vi "Main Page.vi"(8 "error in (no error)":errorcluster, 11 "Node Ptr":T1 format="%.0x") -> (0 "error out":errorcluster)   [LabVIEW 2019, in "FPGA Addon System Explorer.lvlib"]
uses:
  FPGA Addon System Explorer.lvlib
  <vilib>/NI VeriStand/Custom Device API/Custom Device API.lvlib
  Addon Shared/FPGA Addon Shared.lvlib
  Addon Shared/Types/FG Action.ctl
  <vilib>/NI/NI VeriStand Hardware Resource Discovery/NIVS Hardware Discovery.lvlib
  <vilib>/NI/NI VeriStand Hardware Resource Discovery/_Types/Filter Type.ctl
  <vilib>/NI VeriStand/Custom Device API/Custom Device Item Ref.ctl
panel:
  in  "RIO Browse":bool
  out "Version":string
  in  "SHDocVw.IWebBrowser":refnum<k7>(container)
  in  "RIO Device":string
  in  "Bitfile path":path
  in  "Header 2":cluster{"Section Name":string}={"Section Name"="Custom Device Item Settings"}
  in  "Header":cluster{"Section Name":string}={"Section Name"="Custom Device Item Settings"}
  in  "Description":string
  in  "Name":string
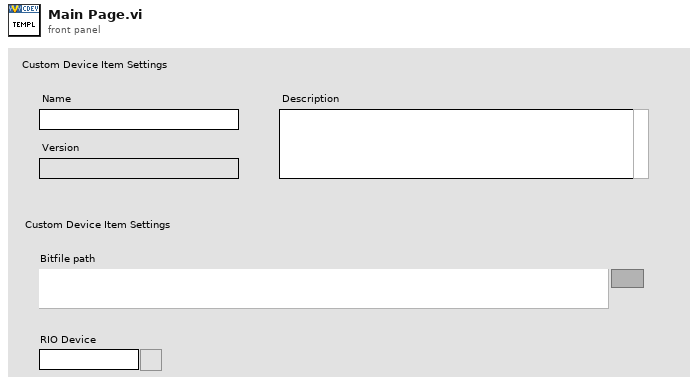
[diagram p1: front panel]
types:
  T1 = typedef "Custom Device API.lvlib/Custom Device Item Ref.ctl" = u64
  T2 = typedef "FPGA Addon Shared.lvlib/FG Action.ctl" = enum8{"GET", "SET"}
  T3 = typedef "FPGA Addon Shared.lvlib/FPGA Settings.ctl" = cluster{"Bitfile path":path, "RIO Device Address":string}
  T4 = typedef "Custom Device API.lvlib/Custom Device Item Info.ctl" = cluster{"Name":string, "Is Channel":bool, "GUID":string, "Is Waveform":bool}
  T5 = typedef "NIVS Hardware Discovery.lvlib/Filter Type.ctl" = enum16{"Device Category", "Product Name", "Ethernet", "XNET", "VISA", "FPGA", "EtherCAT Master", "DAQmx", "GPIB", "Serial"}
  T6 = typedef "Custom Device API.lvlib/Custom Device Commands.ctl" = enum16{"Default", "Item renamed", "Shutdown", "Dynamic button pressed"}
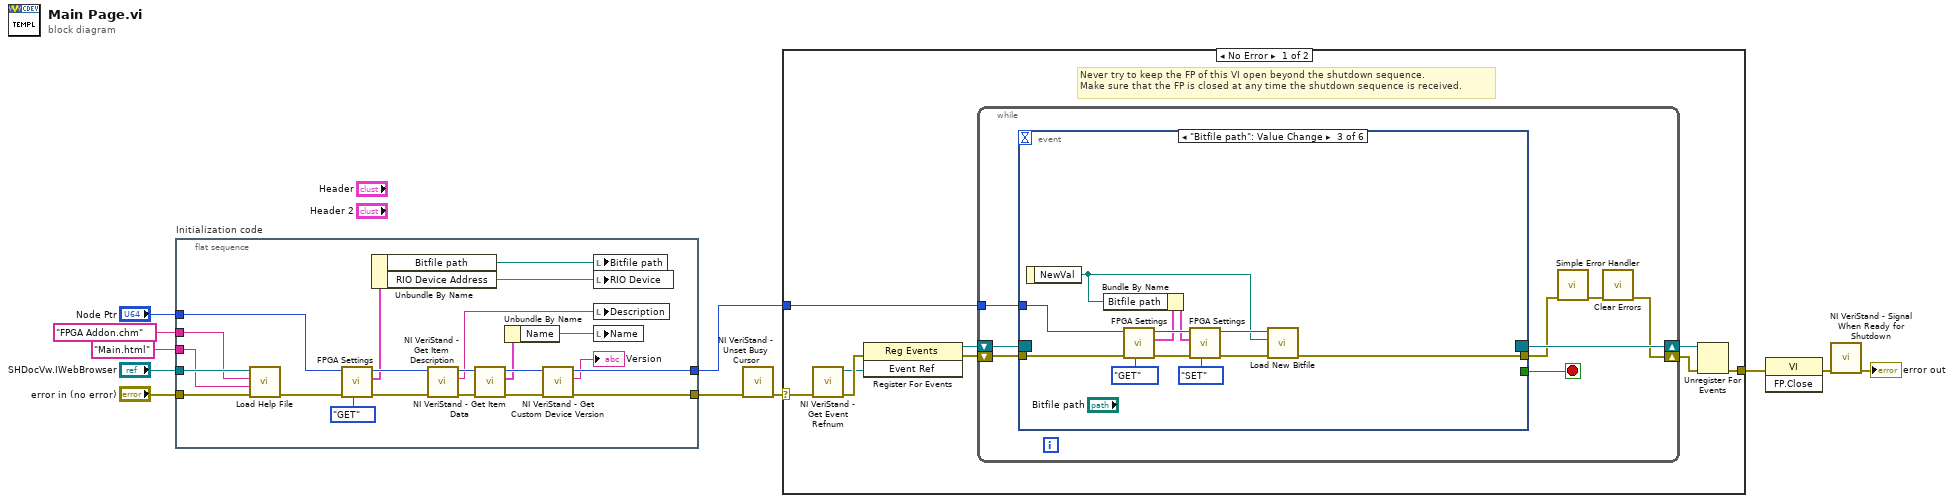
[diagram p0: block diagram]
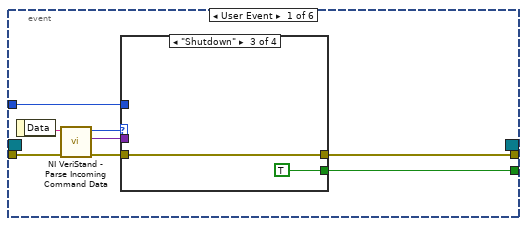
[diagram p2: hidden frame]
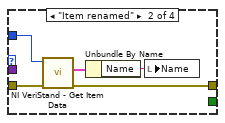
[diagram p4: hidden frame]
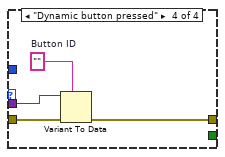
[diagram p5: hidden frame]
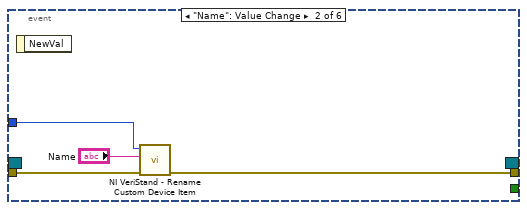
[diagram p6: hidden frame]
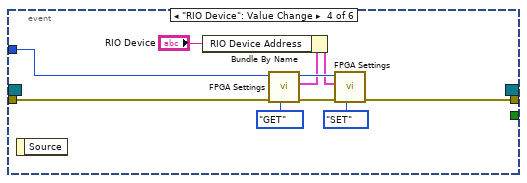
[diagram p7: hidden frame]
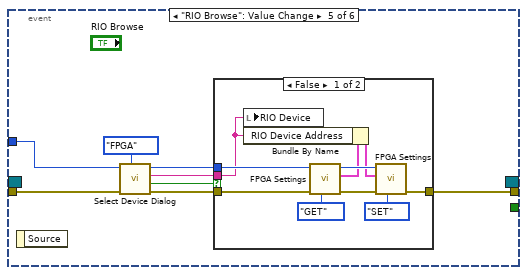
[diagram p8: hidden frame]
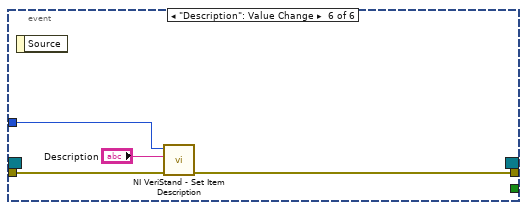
[diagram p10: hidden frame]
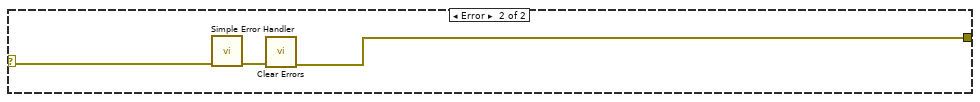
[diagram p11: hidden frame]
diagram:
  n1 = flat-sequence "Initialization code" {
    tunnel: "error in (no error)" -> [w27]
    tunnel: "Node Ptr" -> [w23]
    tunnel: [w14] -> w7
    tunnel: [w15] -> w4
    tunnel: "SHDocVw.IWebBrowser" -> [w26]
    tunnel: "Main.html" ("HTML File") -> [w25]
    tunnel: "FPGA Addon.chm" ("Main CHM File") -> [w24]
    frame #0 {
      n2 = call "Load Help File.vi"("error in (no error)"=w27, "HTML File"=w25, "Main CHM File"=w24, "SHDocVw.IWebBrowser2"=w26) -> ("error out"=w22:errorcluster)  [unwired: 7 in]
      n3 = call "FPGA Settings.vi"("Action"=FG_Action."GET", "error in (no error)"=w22, "Item Ref"=w23) -> ("error out"=w20:errorcluster, "FPGA Settings"=w18:T3, "Item Ref out"=w21:T1)  [unwired: 6 in]
      n4 = Unbundle By Name(w18) -> ("Bitfile path"=w16:path, "RIO Device Address"=w17:string)
      n5 = call <vilib>:"NI VeriStand - Get Item Description.vi"("error in (no error)"=w20, "Item Ref in"=w21) -> ("error out"=w30:errorcluster, "Description"=w31:string, "Item Ref out"=w32:T1)  [unwired: 7 out]
      n6 = call <vilib>:"NI VeriStand - Get Item Data.vi"("error in (no error)"=w30, "Item Ref in"=w32) -> ("error out"=w13:errorcluster, "Item Info"=w29:T4, "Item Ref out"=w33:T1)  [unwired: 7 out]
      n7 = Unbundle By Name(w29) -> ("Name"=w28:string)
      n8 = call <vilib>:"NI VeriStand - Get Custom Device Version.vi"("error in (no error)"=w13, "Device Ref in"=w33) -> ("error out"=w14:errorcluster, "Value"=→"Version":string, "Device Ref out"=w15:T1)  [unwired: 7 in]
      n9 = local write "Bitfile path"(w16) -> ()
      n10 = local write "RIO Device"(w17) -> ()
      n11 = local write "Description"(w31) -> ()
      n12 = local write "Name"(w28) -> ()
    }
  }
  n13 = call <vilib>:"NI VeriStand - Unset Busy Cursor.vi"("error in (no error)"=w7) -> ("error out"=w6:errorcluster)  [unwired: 10 out]
  n14 = case shown="No Error" w6 {
    selector: w6 -> [w34 w122]
    tunnel: [w39 w120] -> w11
    tunnel: w4 -> [w35 _]
    frame No Error {
      # "Never try to keep the FP of this VI open beyond the shutdown sequence.\nMake sure that the FP is closed at any time the shutdown sequence is received."
      n15 = call <vilib>:"NI VeriStand - Get Event Refnum.vi"("error in (no error)"=w34) -> ("error out"=w42:errorcluster, "Event Ref"=w38:refnum<user-event>)  [unwired: 9 out]
      n16 = register-events(error in=w42, w38) -> (reference out=w36:refnum<event-registration>, error out=w37:errorcluster)  [unwired: 1 in]
      n17 = while {
        tunnel: w35 -> [w46]
        shift-right: [w43] -> w40
        shift-left: w37 -> [w49]
        shift-right: [w50] -> w41
        shift-left: w36 -> [w48]
        stop <- w47 stop-if-true
        n18 = event shown="[2] \"Bitfile path\": Value Change" {
          selector: w48 -> [_ _ _ _ _ _]
          dyn-events: [_ _ _ _ _ _] -> w50
          timeout: _ -> [_ _ _ _ _ _]
          tunnel: w49 -> [w58 w74 w81 w90 w102 w118]
          tunnel: [w54 _ _ _ _ _] -> w47
          tunnel: [w53 w73 w86 w87 w104 w117] -> w45
          tunnel: w46 -> [w52 w72 w79 w89 w103 w119]
          event User Event {
            n19 = event-data() -> ("Data"=w57:string)  [unwired: 1 out]
            n20 = call <vilib>:"NI VeriStand - Parse Incoming Command Data.vi"("error in (no error)"=w58, "Incoming data"=w57) -> ("error out"=w56:errorcluster, "Outgoing data"=w51:variant, "Action"=w55:T6)  [unwired: 7 out]
            n21 = case shown="\"Shutdown\"" w55 {
              tunnel: w56 -> [w59 w64 w65 w70]
              tunnel: [_ _ TRUE _] -> w54
              tunnel: [w59 w61 w65 w67] -> w53
              tunnel: w52 -> [_ w63 _ _]
              tunnel: w51 -> [_ _ _ w69]
              frame "Default", Default {
              }
              frame "Item renamed" {
                n22 = call <vilib>:"NI VeriStand - Get Item Data.vi"("error in (no error)"=w64, "Item Ref in"=w63) -> ("error out"=w61:errorcluster, "Item Info"=w62:T4)  [unwired: 8 out]
                n23 = Unbundle By Name(w62) -> ("Name"=w60:string)
                n24 = local write "Name"(w60) -> ()
              }
              frame "Shutdown" {
              }
              frame "Dynamic button pressed" {
                w68 = ""  # Button ID
                n25 = Variant To Data(error in=w70, type=w68, Variant=w69) -> (error out=w67:errorcluster)  [unwired: 1 out]
              }
            }
          }
          event "Name": Value Change {
            n26 = event-data() -> ()  [unwired: 2 out]
            n27 = call <vilib>:"NI VeriStand - Rename Custom Device Item.vi"("error in (no error)"=w74, "New Name"="Name", "Item Ref in"=w72) -> ("error out"=w73:errorcluster)  [unwired: 1 in, 7 out]
          }
          event "Bitfile path": Value Change {
            n28 = event-data() -> ("NewVal"=w75:path)  [unwired: 1 out]
            n29 = call "FPGA Settings.vi"("Action"=FG_Action."GET", "error in (no error)"=w81, "Item Ref"=w79) -> ("error out"=w82:errorcluster, "FPGA Settings"=w77:T3, "Item Ref out"=w83:T1)  [unwired: 6 in]
            n30 = Bundle By Name(cluster=w77, "Bitfile path"=w75) -> (w76:T3)
            n31 = call "FPGA Settings.vi"("Action"=FG_Action."SET", "error in (no error)"=w82, "FPGA Settings"=w76, "Item Ref"=w83) -> ("error out"=w80:errorcluster, "Item Ref out"=w78:T1)  [unwired: 5 in, 1 out]
            n32 = call "Load New Bitfile.vi"("error in (no error)"=w80, "NewVal"=w75, "Item Ref in"=w78) -> ("error out"=w86:errorcluster)  [unwired: 7 in, 1 out]
          }
          event "RIO Device": Value Change {
            n33 = event-data() -> ()  [unwired: 2 out]
            n34 = call "FPGA Settings.vi"("Action"=FG_Action."GET", "error in (no error)"=w90, "Item Ref"=w89) -> ("error out"=w93:errorcluster, "FPGA Settings"=w92:T3, "Item Ref out"=w94:T1)  [unwired: 6 in]
            n35 = Bundle By Name(cluster=w92, "RIO Device Address"="RIO Device") -> (w91:T3)
            n36 = call "FPGA Settings.vi"("Action"=FG_Action."SET", "error in (no error)"=w93, "FPGA Settings"=w91, "Item Ref"=w94) -> ("error out"=w87:errorcluster)  [unwired: 5 in, 2 out]
          }
          event "RIO Browse": Value Change {
            n37 = event-data() -> ()  [unwired: 2 out]
            n38 = call <vilib>:"Select Device Dialog.vi"("Filter Type"=Filter_Type."FPGA", "error in (no error)"=w102, "Item Ref in"=w103) -> ("error out"=w100:errorcluster, "Cancelled?"=w99:bool, "Selected Alias"=w98:string, "Item Ref out"=w101:T1)  [unwired: 5 in]
            n39 = case shown="False" w99 {
              tunnel: w100 -> [w108 w115]
              tunnel: w101 -> [w107 _]
              tunnel: [w106 w115] -> w104
              tunnel: w98 -> [w105 _]
              frame False {
                n40 = local write "RIO Device"(w105) -> ()
                n41 = call "FPGA Settings.vi"("Action"=FG_Action."GET", "error in (no error)"=w108, "Item Ref"=w107) -> ("error out"=w111:errorcluster, "FPGA Settings"=w110:T3, "Item Ref out"=w112:T1)  [unwired: 6 in]
                n42 = Bundle By Name(cluster=w110, "RIO Device Address"=w105) -> (w109:T3)
                n43 = call "FPGA Settings.vi"("Action"=FG_Action."SET", "error in (no error)"=w111, "FPGA Settings"=w109, "Item Ref"=w112) -> ("error out"=w106:errorcluster)  [unwired: 5 in, 2 out]
              }
              frame True {
              }
            }
          }
          event "Description": Value Change {
            n44 = event-data() -> ()  [unwired: 2 out]
            n45 = call <vilib>:"NI VeriStand - Set Item Description.vi"("error in (no error)"=w118, "Description"="Description", "Item Ref in"=w119) -> ("error out"=w117:errorcluster)  [unwired: 8 out]
          }
        }
        n46 = call <vilib>:"Simple Error Handler.vi"("error in (no error)"=w45) -> ("error out"=w44:errorcluster)  [unwired: 1 in, 7 out]
        n47 = call <vilib>:"Clear Errors.vi"("error in (no error)"=w44) -> ("error out"=w43:errorcluster)  [unwired: 1 in, 5 out]
      }
      n48 = Unregister For Events(event registration refnum=w41, error in=w40) -> (error out=w39:errorcluster)
    }
    frame Error {
      n49 = call <vilib>:"Simple Error Handler.vi"("error in (no error)"=w122) -> ("error out"=w121:errorcluster)  [unwired: 1 in, 7 out]
      n50 = call <vilib>:"Clear Errors.vi"("error in (no error)"=w121) -> ("error out"=w120:errorcluster)  [unwired: 1 in, 5 out]
    }
  }
  n51 = invoke class="VI" method="FP.Close"(error in=w11) -> (error out=w10:errorcluster)  [unwired: 2 in, 2 out]
  n52 = call <vilib>:"NI VeriStand - Signal When Ready for Shutdown.vi"("error in (no error)"=w10) -> ("error out"=→"error out":errorcluster)  [unwired: 10 out]
